vi "Emergency Process Stop.vi"(0 "Emergency Process Stop":refnum<vi>, 1 "Start Stop Reactor Array":refnum<vi>, 2 "Reactor Name":string=" and close valves: ", 3 "Reactor Selector":T1(ring), 5 "Current Valve State":refnum<vi>, 7 "System Queue":refnum<vi>, 9 "System JSON Queue":refnum<vi>, 12 "Pump Valves":i32[](array[numeric]), 13 "Debug Mode":refnum<vi>, 14 "Stop Program":refnum<vi>) -> ()   [LabVIEW 2022 SP3]
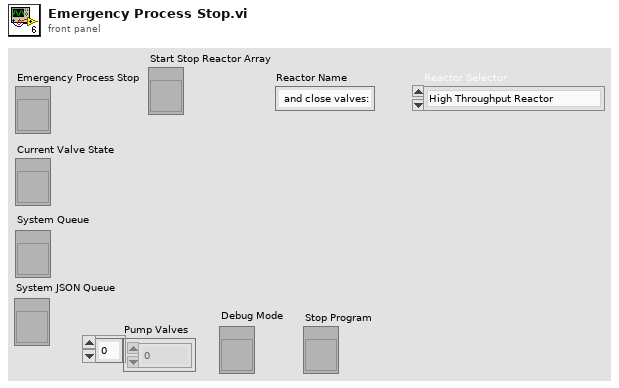
[diagram p1: front panel]
types:
  T1 = enum16{"High Throughput Reactor", "In Situ Reactor", "MLD Reactor"}
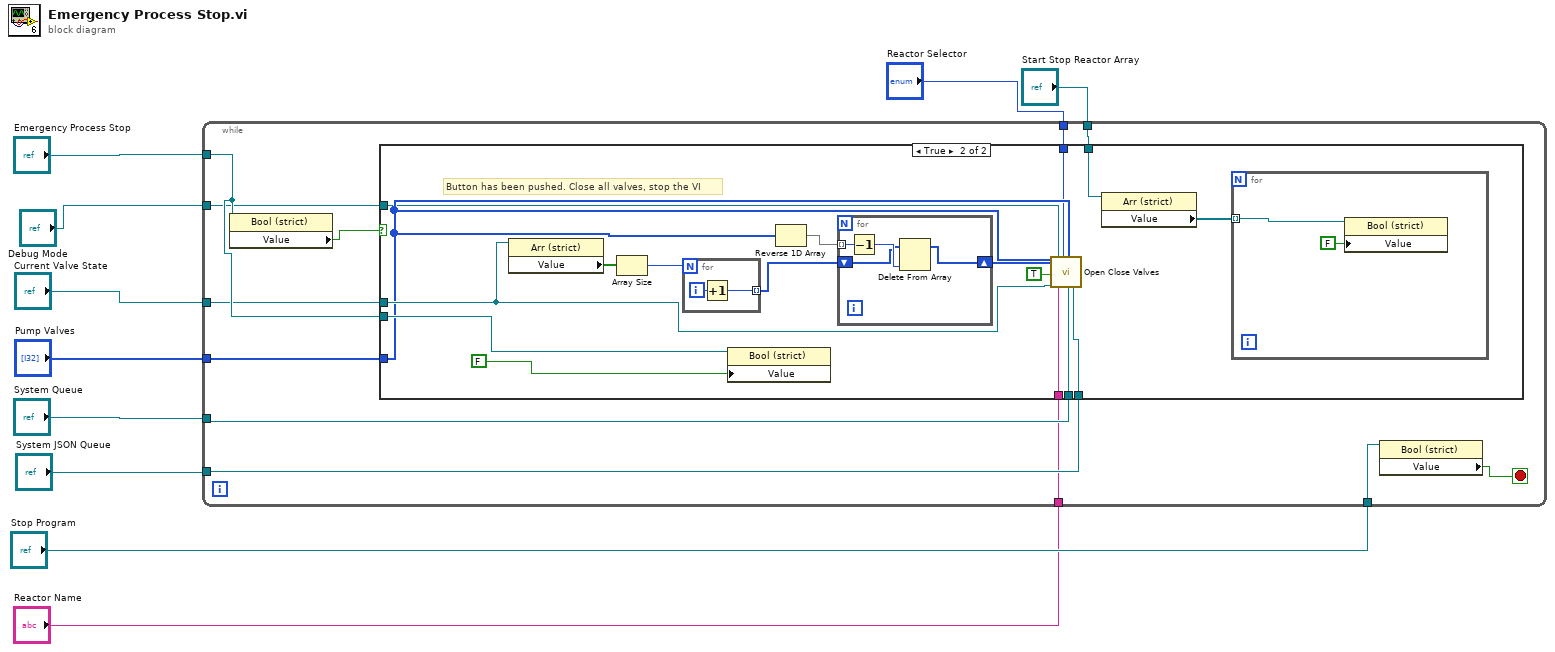
[diagram p0: block diagram]
diagram:
  n1 = while {
    tunnel: "Emergency Process Stop" -> [w21]
    tunnel: "Current Valve State" -> [w20]
    tunnel: "Pump Valves" -> [w19]
    tunnel: "System Queue" -> [w18]
    tunnel: "System JSON Queue" -> [w17]
    tunnel: "Debug Mode" -> [w16]
    tunnel: "Stop Program" -> [w14]
    tunnel: "Start Stop Reactor Array" -> [w13]
    tunnel: "Reactor Name" -> [w12]
    tunnel: "Reactor Selector" -> [w11]
    stop <- w15 stop-if-true
    n2 = property class="Bool (strict)"(reference=w21) -> ("Value"=w22:bool)  [unwired: 1 in, 2 out]
    n3 = case shown="True" w22 {
      tunnel: w21 -> [_ w32]
      tunnel: w20 -> [_ w31]
      tunnel: w19 -> [_ w30]
      tunnel: w18 -> [_ w29]
      tunnel: w17 -> [_ w28]
      tunnel: w16 -> [_ w27]
      tunnel: w13 -> [_ w26]
      tunnel: w12 -> [_ w24]
      tunnel: w11 -> [_ w23]
      frame False {
        # "Button has not been pushed. Do nothing."
      }
      frame True {
        # "Button has been pushed. Close all valves, stop the VI"
        n4 = property class="Arr (strict)"(reference=w31) -> ("Value"=w39:bool[])  [unwired: 1 in, 2 out]
        n5 = Array Size(array=w39) -> (size(s)=w38:i32)
        n6 = for {
          N: w38 -> [_]
          tunnel: [w42] -> w37 mode=indexing
          i -> [w43]
          n7 = Increment(x=w43) -> (x+1=w42:i32)
        }
        n8 = property class="Bool (strict)"(reference=w32, "Value"=FALSE ("Emergency Process Stop")) -> ()  [unwired: 1 in, 2 out]
        n9 = Reverse 1D Array(array=w30) -> (reversed array=w34:i32[])
        n10 = for {
          tunnel: w34 -> [w47] mode=indexing
          shift-right: [w44] -> w36
          shift-left: w37 -> [w45]
          n11 = Decrement(x=w47) -> (x-1=w46:i32)
          n12 = Delete From Array(array=w45, index=w46) -> (array with subset deleted=w44:i32[])  [unwired: 1 in, 1 out]
        }
        n13 = call "Open Close Valves.vi"("Valves to Open"=w30, "Valves to Close"=w36, "Emergency Stop"=TRUE ("stop"), "Current Valve State"=w31, "Debug Mode"=w27, "Reactor Name"=w24, "Reactor Selector"=w23, "Pump Valves"=w30, "System Queue"=w29, "JSON Queue"=w28) -> ()  [unwired: 10 in]
        n14 = property class="Arr (strict)"(reference=w26) -> ("Value"=w25:refnum<vi>[])  [unwired: 1 in, 2 out]
        n15 = for {
          tunnel: w25 -> [w41] mode=indexing
          n16 = property class="Bool (strict)"(reference=w41, "Value"=FALSE) -> ()  [unwired: 1 in, 2 out]
        }
      }
    }
    n17 = property class="Bool (strict)"(reference=w14) -> ("Value"=w15:bool)  [unwired: 1 in, 2 out]
  }
